vi "RFmxSpecAn PreTest Setup.vi"(4 "Frequency (Hz)":dbl=10000000.0 format="%.6p", 6 "Frequency Source":string(combo)="OnboardClock", 8 "error in (no error)":errorcluster, 10 "Reference Level (dBm)":dbl, 11 "Instrument Handle In":refnum<k21>) -> (0 "error out":errorcluster, 3 "Instrument Handle out":refnum<k21>)   [LabVIEW 2018]
uses:
  <vilib>/RFmx/SpecAn/mx/RFmxSpecAn.llb/RFmxSpecAn Select Measurement (Single).vi
  <resource>/objmgr/RFmxSpecAn.rc
  <resource>/objmgr/RFmxInstr.rc
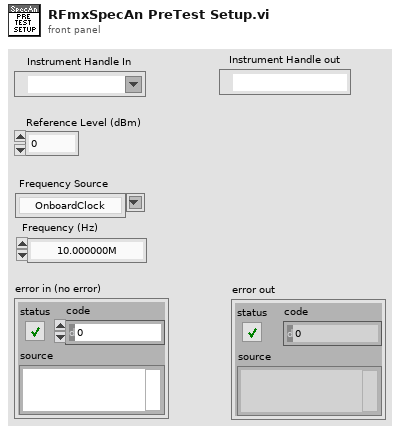
[diagram p1: front panel]
types:
  T1 = enum16{"ACP", "CCDF", "CHP", "FCnt", "Harmonics", "OBW", "SEM", "Spectrum", "Spur", "TXP", "AMPM", "DPD", "IQ", "IM", "NF", "PhaseNoise"}
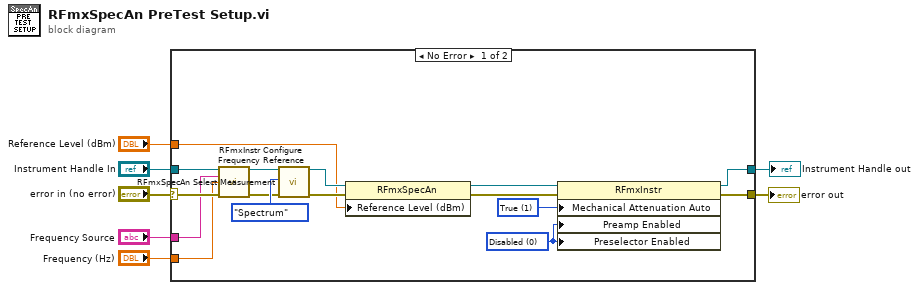
[diagram p0: block diagram]
diagram:
  n1 = case shown="No Error" "error in (no error)" {
    selector: "error in (no error)" -> [w10 w25]
    tunnel: [w16 w25] -> w6
    tunnel: "Reference Level (dBm)" -> [w15 _]
    tunnel: "Instrument Handle In" -> [w11 w24]
    tunnel: [w14 w24] -> w3
    tunnel: "Frequency Source" -> [w9 _]
    tunnel: "Frequency (Hz)" -> [w8 _]
    frame No Error {
      w20 = 0 items=["Disabled"=0, "Enabled"=1, "Automatic"=3] ("Preamp Enabled")
      w17 = 1 items=["False", "True"] ("Mechanical Attenuation Auto")
      n2 = call <vilib>:"RFmxInstr Configure Frequency Reference.vi"("Instrument Handle In"=w11, "Frequency Reference Source"=w9, "Frequency (Hz)"=w8, "error in (no error)"=w10) -> ("Instrument Handle Out"=w13:refnum<k21>, "error out"=w12:errorcluster)  [unwired: 10 in]
      n3 = call-poly <vilib>:"RFmxSpecAn Select Measurement.vi"("Instrument Handle In"=w13, "Measurement"=T1."Spectrum", "error in (no error)"=w12) -> ("Instrument Handle Out"=w18:refnum<k21>, "error out"=w19:errorcluster)  [unwired: 11 in]
      n4 = property class="RFmxSpecAn"(reference=w18, error in=w19, "Reference Level (dBm)"=w15) -> (reference out=w21:refnum<k21>, error out=w22:errorcluster)
      n5 = property class="RFmxInstr"(reference=w21, error in=w22, "Mechanical Attenuation Auto"=w17, "Preamp Enabled"=w20, "Preselector Enabled"=w20) -> (reference out=w14:refnum<k21>, error out=w16:errorcluster)
    }
    frame Error {
    }
  }
  "error out" <- w6
  "Instrument Handle out" <- w3
